vi "remove quotes.vi"(8 "error in (no error)":errorcluster, 11 "string":string) -> (0 "error out":errorcluster, 2 "in quotes?":bool, 3 "without quotes":string)   [LabVIEW 2024, in "controls manager.lvlib"]
uses:
  controls manager.lvlib
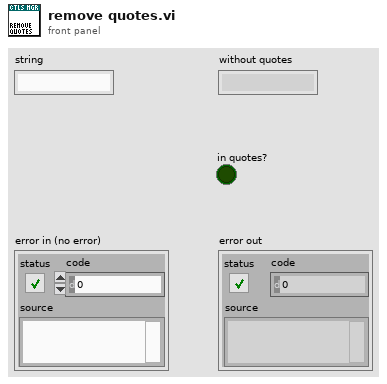
[diagram p1: front panel]
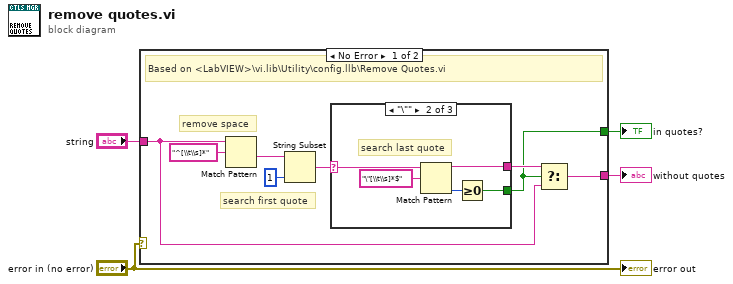
[diagram p0: block diagram]
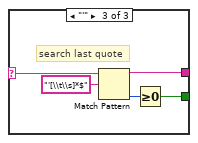
[diagram p3: hidden frame]
diagram:
  n1 = case shown="No Error" "error in (no error)" {
    tunnel: [w6 w23] -> w4
    tunnel: "string" -> [w7 w23]
    tunnel: [w5 _] -> w3
    frame No Error {
      # "remove space"
      # "search first quote"
      # "Based on <LabVIEW>\\vi.lib\\Utility\\config.llb\\Remove Quotes.vi"
      n2 = Match Pattern(string=w7, regular expression="^[\\t\\s]*") -> (after substring=w12:string)  [unwired: 1 in, 3 out]
      n3 = String Subset(string=w12, length (rest)=1) -> (substring=w10:string)  [unwired: 1 in]
      n4 = case shown="\"\\\"\"" w10 {
        selector: w10 -> [_ w13 w18]
        tunnel: [_ w16 w20] -> w5
        tunnel: [_ w15 w21] -> w11
        frame Default {
        }
        frame "\"" {
          # "search last quote"
          n5 = Match Pattern(string=w13, regular expression="\"[\\t\\s]*$") -> (before substring=w15:string, offset past match=w14:i32)  [unwired: 1 in, 2 out]
          n6 = Greater Or Equal To 0?(x=w14) -> (x >= 0?=w16:bool)
        }
        frame "'" {
          # "search last quote"
          n7 = Match Pattern(string=w18, regular expression="'[\\t\\s]*$") -> (before substring=w21:string, offset past match=w19:i32)  [unwired: 1 in, 2 out]
          n8 = Greater Or Equal To 0?(x=w19) -> (x >= 0?=w20:bool)
        }
      }
      n9 = Select(t=w11, s=w5, f=w7) -> (s? t:f=w6:string)
    }
    frame Error {
    }
  }
  "without quotes" <- w4
  "in quotes?" <- w3
  "error out" <- "error in (no error)"
